vi "Get value by Variant.vi"(8 "error in (no error)":errorcluster, 11 "Column Parent in":refnum<class "Column Parent.lvclass">) -> (0 "error out":errorcluster, 2 "Variant":variant, 3 "Column Parent out":refnum<class "Column Parent.lvclass">)   [LabVIEW 2020, in "Basic Columns.lvlib" / "Column Parent.lvclass"]
uses:
  Column Parent.lvclass
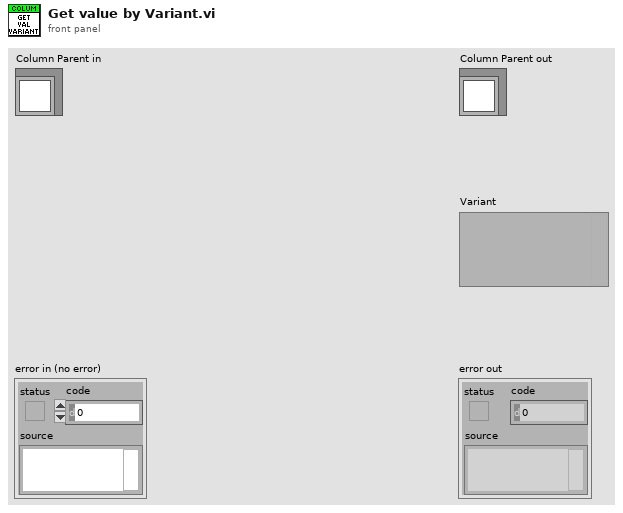
[diagram p1: front panel]
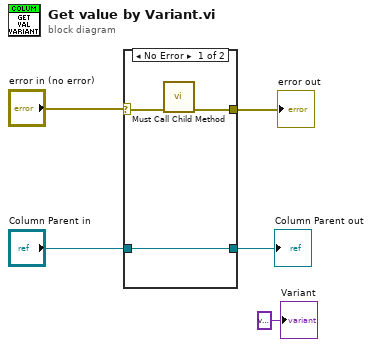
[diagram p0: block diagram]
diagram:
  n1 = case shown="No Error" "error in (no error)" {
    selector: "error in (no error)" -> [w7 w10]
    tunnel: [w6 w10] -> w3
    tunnel: "Column Parent in" -> [w8 w9]
    tunnel: [w8 w9] -> w1
    frame No Error {
      n2 = call "Must Call Child Method.vi"("error in"=w7) -> ("error out"=w6:errorcluster)  [unwired: 10 in]
    }
    frame Error {
    }
  }
  "error out" <- w3
  "Column Parent out" <- w1
  "Variant" <- variant ("Variant")
